vi "GdsLanguage_Init.vi"(0 "PrimaryLanguage":T1=enum."en", 2 "LanguageFilesDirectory(Use current if not wired)":path, 4 "ChesumControl":T2, 5 "error in (no error)":errorcluster) -> (15 "FoundLanguages":T1[](array[typedef]), 17 "NoOfLangaugeStrings":i32, 18 "NoOfLanuageStringsCurrentLanguageHas":i32, 19 "error out":errorcluster)   [LabVIEW 2014]
doc: "Sets the current and backup languages, validates these languages (checks that \nthere are non-empty strings for all StringID entries), and load the translated strings into class memory for later use in the application."
uses:
  <resource>/Framework/Providers/Open_GDS/ClassProviders/Common/GdsLanguage/GdsLanguage_LanguageID.ctl
  <resource>/Framework/Providers/Open_GDS/ClassProviders/Common/GdsLanguage/private/GdsLanguage_ChecksumCheckType.ctl
  <resource>/Framework/Providers/Open_GDS/SubVIs/GOOP_ErrorCodes.ctl
panel:
  out "DuplicateTranslations":string[](array[string])
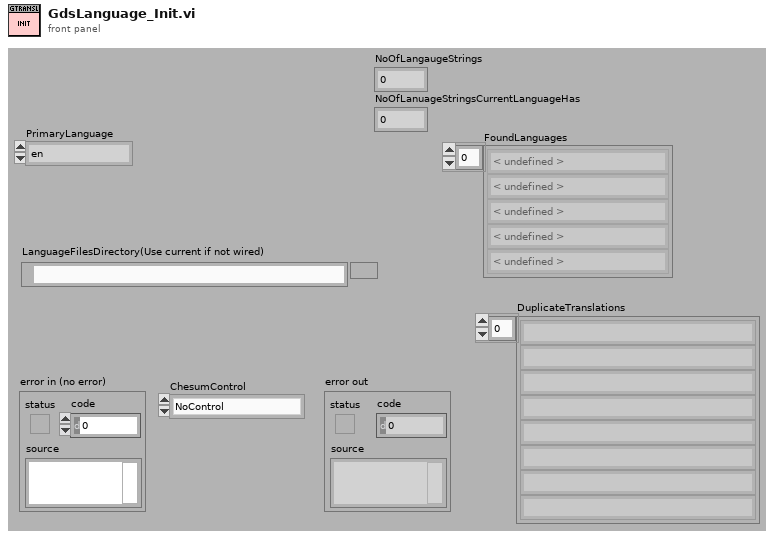
[diagram p1: front panel]
types:
  T1 = typedef "GdsLanguage_LanguageID.ctl" = enum16{"< undefined >", "aa", "ab", "af", "am", "ar", "as", "ay", "az", "ba", "be", "bg", "bh", "bi", "bn", "bo", "br", "ca", "co", "cs", "cy", "da", "de", "dz", "el", "en", "eo", "es", "et", "eu", "fa", "fi", "fj", "fo", "fr", "fy", "ga", "gd", "gl", "gn", "gu", "gv", "ha", "he", "hi", "hr", "hu", "hy", "ia", "id", "ie", "ik", "is", "it", "iu", "ja", "jv", "ka", "kk", "kl", "km", "kn", "ko", "ks", "ku", "ky", "la", "li", "ln", "lo", "lt", "lv", "mg", "mi", "mk", "ml", "mn", "mo", "mr", "ms", "mt", "my", "na", "ne", "nl", "no", "oc", "om", "or", "pa", "pl", "ps", "pt", "qu", "rm", "rn", "ro", "ru", "rw", "sa", "sd", "sg", "sh", "si", "sk", "sl", "sm", "sn", "so", "sq", "sr", "ss", "st", "su", "sv", "sw", "ta", "te", "tg", "th", "ti", "tk", "tl", "tn", "to", "tr", "ts", "tt", "tw", "ug", "uk", "ur", "uz", "vi", "vo", "wo", "xh", "yi", "yo", "zh", "zu"}
  T2 = typedef "GdsLanguage_ChecksumCheckType.ctl" = enum16{"NoControl", "CheckChecksum", "AddChecksum"}
  T3 = typedef "GOOP_ErrorCodes.ctl" = enum16{"LicenseFileMissing", "LicenseFileNotCorrect", "NoProductAccessGranted", "AgreementNoAccepted", "NoValidProviderFound", "LicenseExpired", "LanguageUndefined", "LanguageFileMissing", "LanguageFileChecksumError", "DublicateLanguageTranslation", "LanguageStringIDNotFound", "CommunityLimitReached", "ClassFileLocked", "ClassFileReadOnly", "ProjectNotValid"}
  T4 = typedef "GdsLanguage_ObjectAttributes.ctl" = cluster{"Language":T1, "TranslatedStrings":string[], "StringIDArray":string[], "LanguageFilesDirectory":path, "AvailableLanguages":T1[]}
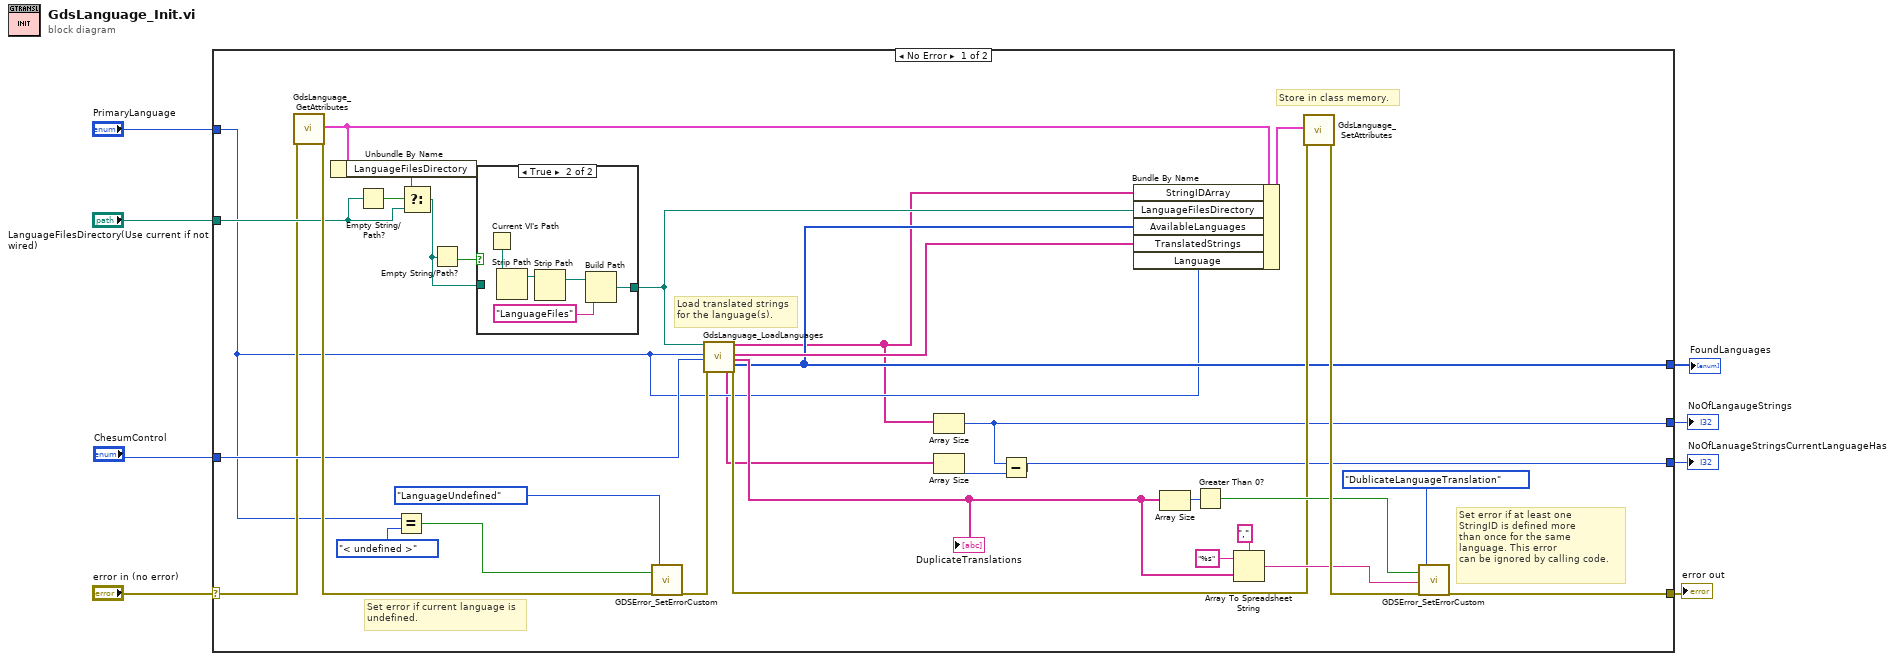
[diagram p0: block diagram]
diagram:
  n1 = case shown="No Error" "error in (no error)" {
    selector: "error in (no error)" -> [w24 w48]
    tunnel: [w20 w48] -> w7
    tunnel: "PrimaryLanguage" -> [w14 _]
    tunnel: "LanguageFilesDirectory(Use current if not wired)" -> [w26 _]
    tunnel: "ChesumControl" -> [w25 _]
    tunnel: [w21 _] -> w3
    tunnel: [w10 _] -> w2
    tunnel: [w11 _] -> w1
    frame No Error {
      # "Set error if at least one\nStringID is defined more\nthan once for the same\nlanguage. This error \ncan be ignored by calling code."
      # "Set error if current language is\nundefined."
      # "Store in class memory."
      # "Load translated strings\nfor the language(s)."
      n2 = call <resource>:"GdsLanguage_GetAttributes.vi"("error in (no error)"=w24) -> ("Attributes"=w29:T4, "error out"=w30:errorcluster)  [unwired: 17 in]
      n3 = Unbundle By Name(w29) -> ("LanguageFilesDirectory"=w27:path)
      n4 = Empty String/Path?(string/path=w26) -> (empty?=w28:bool)
      n5 = Equal?(x=w14, y=GdsLanguage_LanguageID."< undefined >" ("x")) -> (x = y?=w38:bool)
      n6 = Select(t=w27, s=w28, f=w26) -> (s? t:f=w16:path)
      n7 = Empty String/Path?(string/path=w16) -> (empty?=w17:bool)
      n8 = case shown="True" w17 {
        tunnel: w16 -> [w42 _]
        tunnel: [w42 w44] -> w15
        frame False {
        }
        frame True {
          n9 = Current VI's Path() -> (path=w43:path)
          n10 = Strip Path(path=w43) -> (stripped path=w47:path)  [unwired: 1 out]
          n11 = Strip Path(path=w47) -> (stripped path=w46:path)  [unwired: 1 out]
          n12 = Build Path(base path=w46, name or relative path="LanguageFiles") -> (appended path=w44:path)
        }
      }
      n13 = call <resource>:"GDSError_SetErrorCustom.vi"("status"=w38, "error in (no error)"=w30, "UserDefinedCodes(+5000)"=GOOP_ErrorCodes."LanguageUndefined") -> ("error out"=w40:errorcluster)  [unwired: 16 in]
      n14 = call <resource>:"GdsLanguage_LoadLanguages.vi"("LanguageFilesDirectory"=w15, "LanguagesToLoad"=w14, "ChesumControl"=w25, "error in (no error)"=w40) -> ("StringIDsMissingThisLangaugeTranslation"=w12:string[], "StringIDArray"=w13:string[], "TranslatedStrings"=w23:string[], "DuplicateTranslations"=w34:string[], "FoundLanguages"=w21:T1[], "error out"=w31:errorcluster)  [unwired: 10 in]
      "DuplicateTranslations" <- w34
      n15 = Array Size(array=w13) -> (size(s)=w11:i32)
      n16 = Array Size(array=w12) -> (size(s)=w9:i32)
      n17 = Subtract(x=w11, y=w9) -> (x-y=w10:i32)
      n18 = Bundle By Name(cluster=w29, "StringIDArray"=w13, "LanguageFilesDirectory"=w15, "AvailableLanguages"=w21, "TranslatedStrings"=w23, "Language"=w14) -> (w41:T4)
      n19 = Array Size(array=w34) -> (size(s)=w36:i32)
      n20 = Greater Than 0?(x=w36) -> (x > 0?=w35:bool)
      n21 = Array To Spreadsheet String(delimiter (Tab)=",", array=w34, 3:"%s" ("format string")) -> (spreadsheet string=w33:string)
      n22 = call <resource>:"GdsLanguage_SetAttributes.vi"("Attributes"=w41, "error in (no error)"=w31) -> ("error out"=w37:errorcluster)  [unwired: 17 in]
      n23 = call <resource>:"GDSError_SetErrorCustom.vi"("status"=w35, "source"=w33, "error in (no error)"=w37, "UserDefinedCodes(+5000)"=GOOP_ErrorCodes."DublicateLanguageTranslation") -> ("error out"=w20:errorcluster)  [unwired: 15 in]
    }
    frame Error {
    }
  }
  "error out" <- w7
  "FoundLanguages" <- w3
  "NoOfLangaugeStrings" <- w1
  "NoOfLanuageStringsCurrentLanguageHas" <- w2
